vi "FreqResponseSpecCalc.vi"(10 "Freq Response Spec In":cluster{"Freq":dbl, "Upper":dbl, "Lower":dbl}[](array[cluster]), 11 "Freq List In":cluster{"Freq":dbl, "Amp":dbl}[](array[cluster])) -> (2 "All Freq Spec Out":cluster{"Freq":dbl, "Upper":dbl, "Lower":dbl}[](array[cluster]), 3 "XY Graph":cluster{dbl[], dbl[]}[](graph))   [LabVIEW 2018]
panel:
  out "Lower":dbl[](array[numeric])
  out "Upper":dbl[](array[numeric])
  out "Freq":dbl[](array[numeric])
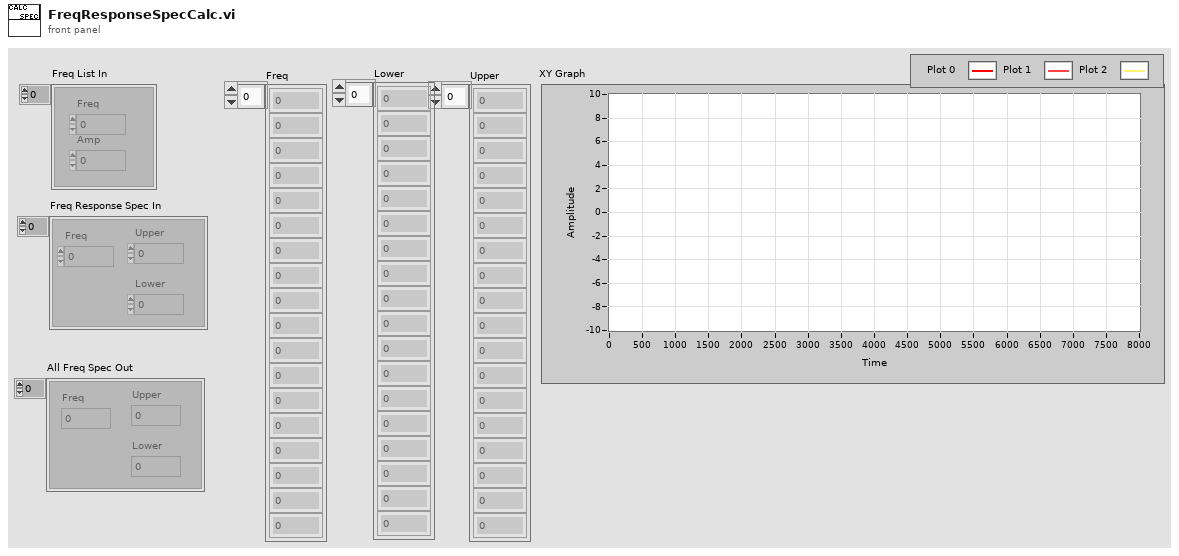
[diagram p1: front panel]
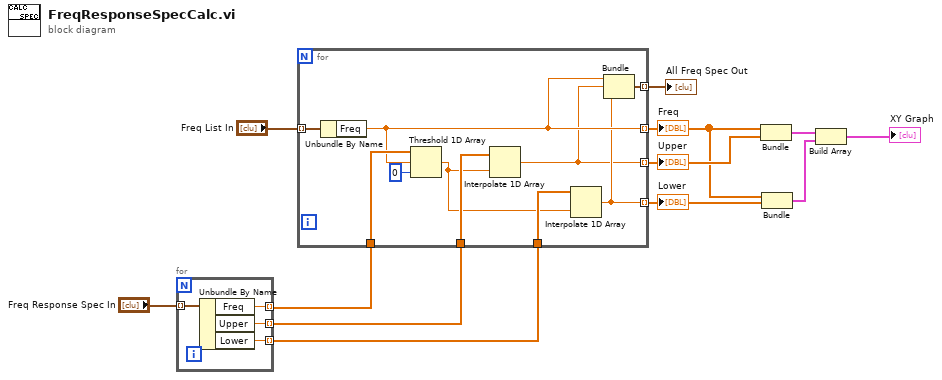
[diagram p0: block diagram]
diagram:
  n1 = for {
    tunnel: "Freq Response Spec In" -> [w16] mode=indexing
    tunnel: [w15] -> w10 mode=indexing
    tunnel: [w14] -> w9 mode=indexing
    tunnel: [w13] -> w8 mode=indexing
    n2 = Unbundle By Name(w16) -> ("Freq"=w15:dbl, "Upper"=w14:dbl, "Lower"=w13:dbl)
  }
  n3 = for {
    tunnel: "Freq List In" -> [w26] mode=indexing
    tunnel: [w20] -> w6 mode=indexing
    tunnel: w10 -> [w25]
    tunnel: w9 -> [w23]
    tunnel: w8 -> [w22]
    tunnel: [w18] -> w7 mode=indexing
    tunnel: [w19] -> w5 mode=indexing
    tunnel: [w17] -> w2 mode=indexing
    n4 = Unbundle By Name(w26) -> ("Freq"=w20:dbl)
    n5 = Threshold 1D Array(1:0 ("start index (0)"), 2:w20, 3:w25) -> (0:w21:dbl)
    n6 = Interpolate 1D Array(1:w21, 2:w23) -> (0:w18:dbl)
    n7 = Interpolate 1D Array(1:w21, 2:w22) -> (0:w19:dbl)
    n8 = Bundle("Freq"=w20, w18, w19) -> (w17:cluster{"Freq":dbl, dbl, dbl})  [unwired: 1 in]
  }
  "Freq" <- w6
  "Upper" <- w7
  "Lower" <- w5
  "All Freq Spec Out" <- w2
  n9 = Bundle(w6, w7) -> (w3:cluster{dbl[], dbl[]})  [unwired: 1 in]
  n10 = Bundle(w6, w5) -> (w4:cluster{dbl[], dbl[]})  [unwired: 1 in]
  n11 = Build Array(w3, w4) -> (→"XY Graph":cluster{dbl[], dbl[]}[])
